vi "resolve control references.vi"(4 "output dictionary":refnum<class "data dictionary.lvclass">, 6 "input dictionary":refnum<class "data dictionary.lvclass">, 8 "error in":errorcluster, 10 "bitfile ref":refnum<k20>, 11 "channels in":refnum<class "TBM channel.lvclass">[](array[class])) -> (0 "error out":errorcluster, 2 "indicators":T1[](array[typedef]), 3 "controls":T1[](array[typedef]))   [LabVIEW 2015, in "io runtime.lvclass"]
uses:
  io runtime.lvclass
  <vilib>/NI/Tag Bus Module Framework/channel/TBM channel.lvclass
  control index set.ctl
  <vilib>/NI/Tag Bus/tag/Data Type.ctl
  configuration/fpga resource supported data types.ctl
  <vilib>/NI/Tag Bus/dictionary/data dictionary.lvclass
  fpga channel/fpga channel.lvclass
  <vilib>/NI/Tag Bus Module Framework/channel/TBM channel.lvclass/TBM channel.ctl
  <vilib>/NI/Tag Bus/tag/tag descriptor.lvclass/tag descriptor.ctl
  <vilib>/NI/Tag Bus Module Framework/channel/Read channel classification.vi
  <vilib>/NI/Tag Bus/tag/read tag name.vi
  <vilib>/NI/Tag Bus/tag/read data type.vi
  <vilib>/NI/Tag Bus/tag/tag descriptor.lvclass
  <vilib>/NI/Configuration Framework/NISE_CEF_TreeControl.lvlib
  configuration/io configuration.lvclass
  <vilib>/NI/LVFPGA Adv Session Resources/LVFPGAAdvSessionResources.lvlib
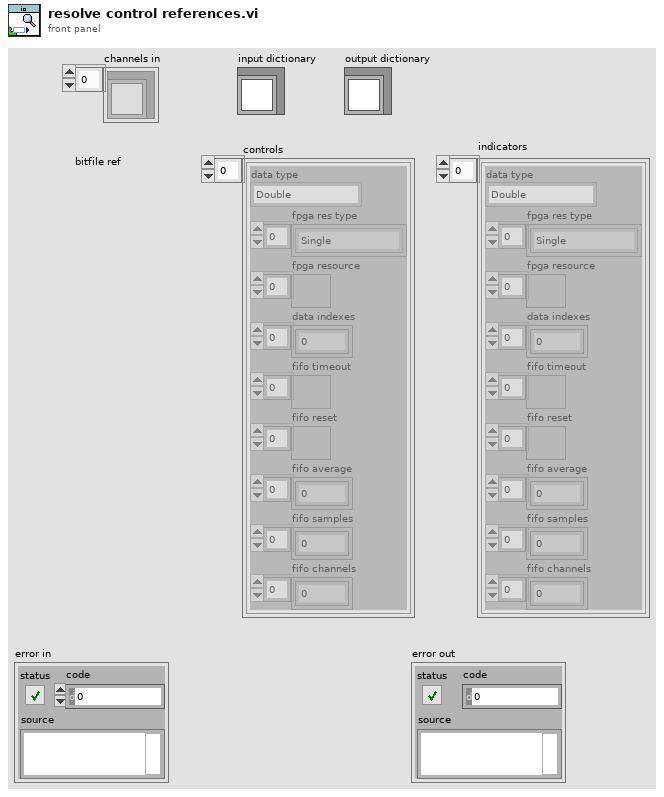
[diagram p1: front panel]
types:
  T1 = typedef "io runtime.lvclass/control index set.ctl" = cluster{"data type":T2, "fpga res type":T3[], "fpga resource":refnum<k20>[], "data indexes":i32[], "fifo timeout":refnum<k20>[], "fifo reset":refnum<k20>[], "fifo average":i32[], "fifo samples":u32[], "fifo channels":u32[]}
  T2 = typedef "tag bus.lvlib/tag descriptor.lvclass/Data Type.ctl" = enum16{"Double", "Single", "I64", "I32", "I16", "I8", "U64", "U32", "U16", "U8", "Boolean", "String", "Array of Double", "Array of Single", "Array of I64", "Array of I32", "Array of I16", "Array of I8", "Array of U64", "Array of U32", "Array of U16", "Array of U8", "Array of Boolean", "Array of String"}
  T3 = typedef "io configuration.lvclass/fpga resource supported data types.ctl" = enum16{"Invalid Type", "Single", "I64", "I32", "I16", "I8", "U64", "U32", "U16", "U8", "Boolean", "FXP I,20,5", "FXP I,24,5", "FXP I,24,10", "Fifo 1023,I16"}
  T4 = typedef "LVFPGAAdvSessionResources.lvlib/ResourceInfo.ctl" = cluster{"Resource name":string, "Data type":variant, "Resource type":enum16{"Register", "Host To Target FIFO", "Target To Host FIFO"}}
  T5 = typedef "TBM channel.lvclass/channel classification.ctl" = enum16{"input data", "output data", "processing parameter", "processing result"}
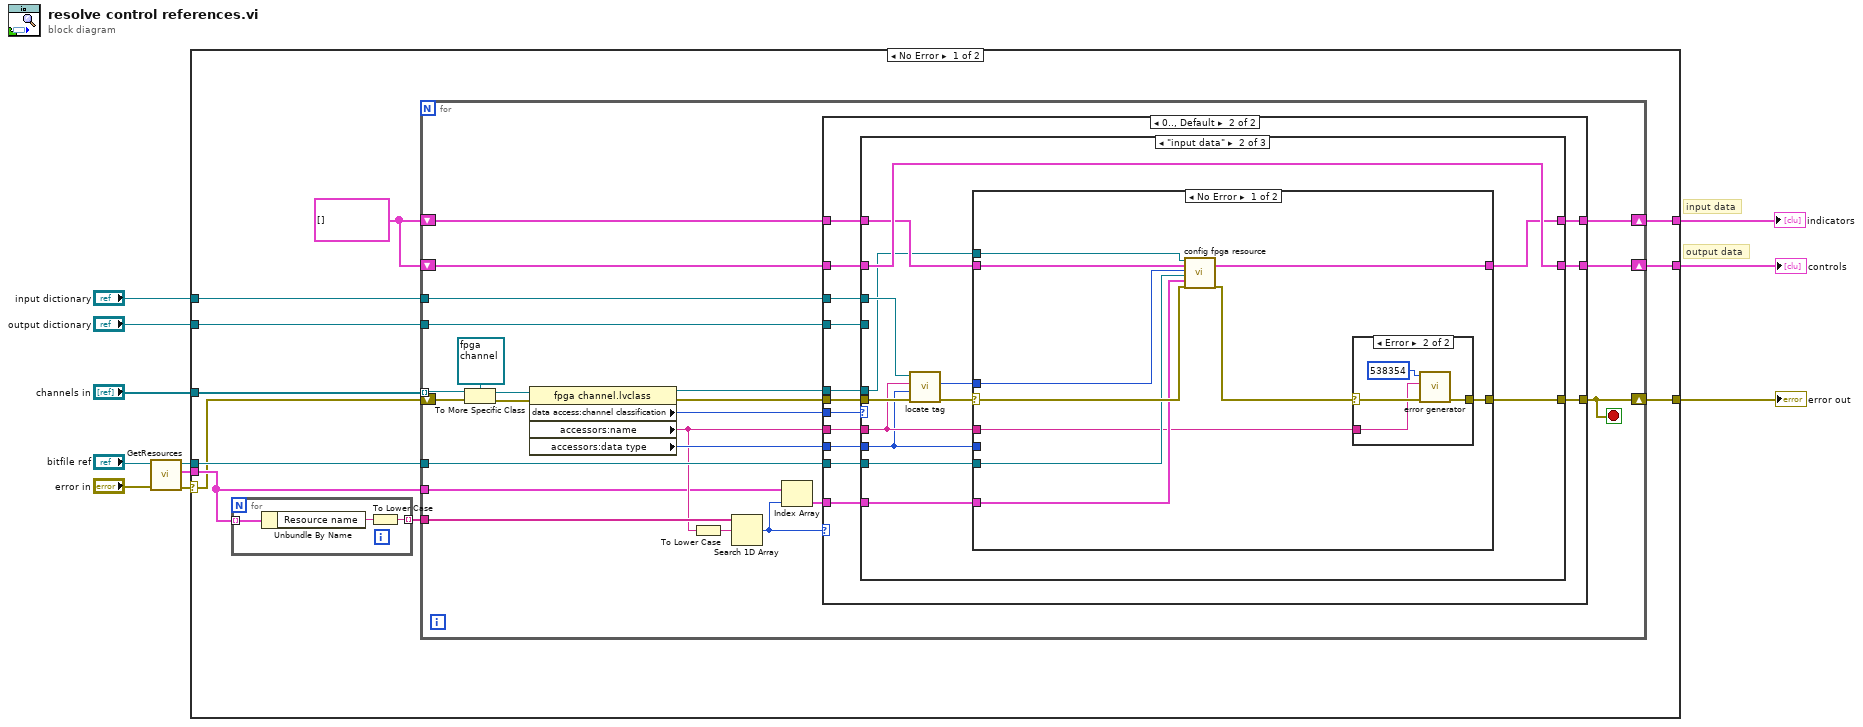
[diagram p0: block diagram]
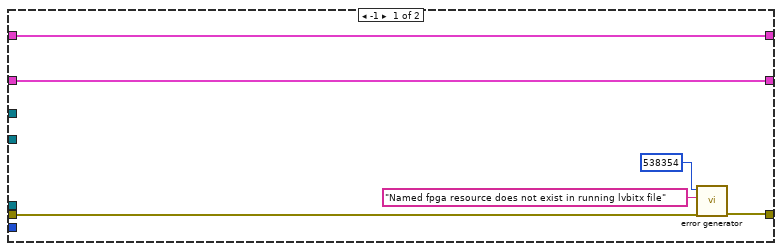
[diagram p2: hidden frame]
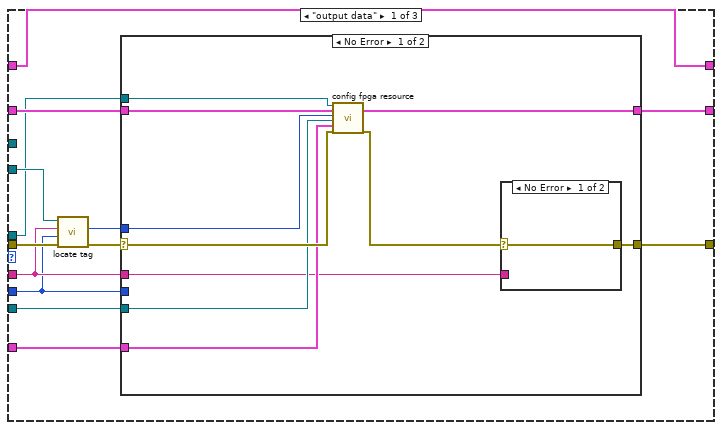
[diagram p3: hidden frame]
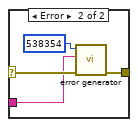
[diagram p4: hidden frame]
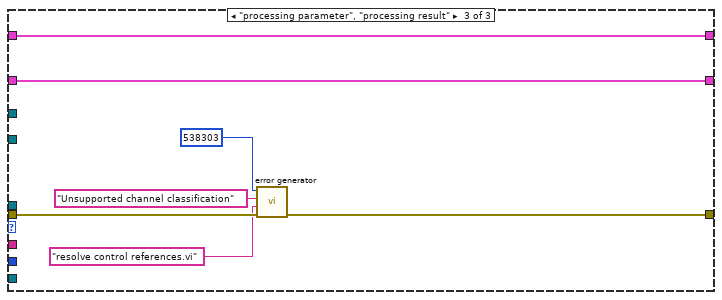
[diagram p8: hidden frame]
diagram:
  # "input data"
  # "output data"
  n1 = call <vilib>:"GetResources.vi"("error in (no error)"="error in", "FPGA VI Reference in"="bitfile ref") -> ("error out"=w1:errorcluster, "Resource info out"=w2:T4[], "FPGA VI Reference out"=w3:refnum<k20>)  [unwired: 7 in]
  n2 = case shown="No Error" w1 {
    selector: w1 -> [w12 w136]
    tunnel: "channels in" -> [w22 _]
    tunnel: [w20 _] -> w6
    tunnel: [w19 _] -> w5
    tunnel: "output dictionary" -> [w18 _]
    tunnel: "input dictionary" -> [w17 _]
    tunnel: [w16 w136] -> w7
    tunnel: w3 -> [w14 _]
    tunnel: w2 -> [w13 _]
    frame No Error {
      w21 = T1[] [] ("indicators")
      n3 = for {
        tunnel: w13 -> [w25] mode=indexing
        tunnel: [w23] -> w15 mode=indexing
        n4 = Unbundle By Name(w25) -> ("Resource name"=w24:string)
        n5 = To Lower Case(string=w24) -> (all lower case string=w23:string)
      }
      n6 = for {
        tunnel: w22 -> [w26] mode=indexing
        shift-right: [w45] -> w20
        shift-left: w21 -> [w44]
        shift-right: [w42] -> w19
        shift-left: w21 -> [w43]
        shift-right: [w46] -> w16
        shift-left: w12 -> [w33]
        tunnel: w18 -> [w40]
        tunnel: w17 -> [w41]
        tunnel: w14 -> [w39]
        tunnel: w15 -> [w36]
        tunnel: w13 -> [w29]
        stop <- w46 stop-if-true
        n7 = To More Specific Class(target class=refnum<class "fpga channel.lvclass"> refnum ("fpga channel.lvclass"), reference=w26, error in=w33) -> (specific class reference=w32:refnum<class "fpga channel.lvclass">, error out=w27:errorcluster)
        n8 = property class="fpga channel.lvclass"(reference=w32, error in=w27) -> (reference out=w37:refnum<class "fpga channel.lvclass">, error out=w47:errorcluster, "data access:channel classification"=w48:T5, "accessors:name"=w35:string, "accessors:data type"=w38:T2)
        n9 = To Lower Case(string=w35) -> (all lower case string=w34:string)
        n10 = Search 1D Array(1D array=w36, element=w34) -> (index of element=w30:i32)  [unwired: 1 in]
        n11 = Index Array(array=w29, index=w30) -> (element=w28:T4)
        n12 = case shown="0.., Default" w30 {
          tunnel: w48 -> [_ w68]
          tunnel: w47 -> [w53 w67]
          tunnel: [w52 w66] -> w46
          tunnel: [w51 w65] -> w45
          tunnel: w44 -> [w51 w64]
          tunnel: w43 -> [w50 w63]
          tunnel: [w50 w62] -> w42
          tunnel: w41 -> [_ w61]
          tunnel: w40 -> [_ w60]
          tunnel: w39 -> [_ w59]
          tunnel: w38 -> [_ w58]
          tunnel: w37 -> [_ w57]
          tunnel: w35 -> [_ w56]
          tunnel: w28 -> [_ w55]
          frame -1 {
            n13 = call <vilib>:"error generator.vi"("error in"=w53, "append error message"="Named fpga resource does not exist in running lvbitx file", "error code (0)"=538354) -> ("error out"=w52:errorcluster)  [unwired: 6 in]
          }
          frame 0.., Default {
            n14 = case shown="\"input data\"" w68 {
              tunnel: w67 -> [w81 w110 w135]
              tunnel: [w77 w106 w133] -> w66
              tunnel: [w71 w100 w130] -> w65
              tunnel: w64 -> [w71 w101 w130]
              tunnel: w63 -> [w73 w111 w129]
              tunnel: [w72 w111 w129] -> w62
              tunnel: w61 -> [_ w102 _]
              tunnel: w56 -> [w79 w108 _]
              tunnel: w58 -> [w78 w107 _]
              tunnel: w60 -> [w74 _ _]
              tunnel: w59 -> [w75 w104 _]
              tunnel: w57 -> [w70 w99 _]
              tunnel: w55 -> [w69 w103 _]
              frame "output data" {
                n15 = call <vilib>:"locate tag.vi"("error in"=w81, "data type"=w78, "name"=w79, "data dictionary in"=w74) -> ("error out"=w80:errorcluster, "index"=w76:i32)  [unwired: 5 in, 1 out]
                n16 = case shown="No Error" w80 {
                  selector: w80 -> [w90 w98]
                  tunnel: w79 -> [w82 _]
                  tunnel: w78 -> [_ _]
                  tunnel: [w91 w98] -> w77
                  tunnel: w73 -> [w87 w97]
                  tunnel: [w86 w97] -> w72
                  tunnel: w76 -> [w85 _]
                  tunnel: w75 -> [w84 _]
                  tunnel: w70 -> [w88 _]
                  tunnel: w69 -> [w83 _]
                  frame No Error {
                    n17 = call-dynamic "config fpga resource.vi"("fpga channel in"=w88, "pairs in"=w87, "tagbus index"=w85, "bitfile ref in"=w84, "hardware resource"=w83, "error in (no error)"=w90) -> ("pairs out"=w86:T1[], "error out"=w89:errorcluster)  [unwired: 11 in, 1 out]
                    n18 = case shown="No Error" w89 {
                      selector: w89 -> [w92 w94]
                      tunnel: [w92 w95] -> w91
                      tunnel: w82 -> [_ w93]
                      frame No Error {
                      }
                      frame Error {
                        n19 = call <vilib>:"error generator.vi"("error in"=w94, "append error message"=w93, "error code (0)"=538354) -> ("error out"=w95:errorcluster)  [unwired: 6 in]
                      }
                    }
                  }
                  frame Error {
                  }
                }
              }
              frame "input data" {
                n20 = call <vilib>:"locate tag.vi"("error in"=w110, "data type"=w107, "name"=w108, "data dictionary in"=w102) -> ("error out"=w109:errorcluster, "index"=w105:i32)  [unwired: 5 in, 1 out]
                n21 = case shown="No Error" w109 {
                  selector: w109 -> [w120 w128]
                  tunnel: w108 -> [w112 _]
                  tunnel: w107 -> [_ _]
                  tunnel: [w121 w128] -> w106
                  tunnel: w101 -> [w117 w127]
                  tunnel: [w116 w127] -> w100
                  tunnel: w105 -> [w115 _]
                  tunnel: w104 -> [w114 _]
                  tunnel: w99 -> [w118 _]
                  tunnel: w103 -> [w113 _]
                  frame No Error {
                    n22 = call-dynamic "config fpga resource.vi"("fpga channel in"=w118, "pairs in"=w117, "tagbus index"=w115, "bitfile ref in"=w114, "hardware resource"=w113, "error in (no error)"=w120) -> ("pairs out"=w116:T1[], "error out"=w119:errorcluster)  [unwired: 11 in, 1 out]
                    n23 = case shown="Error" w119 {
                      selector: w119 -> [w122 w124]
                      tunnel: [w122 w125] -> w121
                      tunnel: w112 -> [_ w123]
                      frame No Error {
                      }
                      frame Error {
                        n24 = call <vilib>:"error generator.vi"("error in"=w124, "append error message"=w123, "error code (0)"=538354) -> ("error out"=w125:errorcluster)  [unwired: 6 in]
                      }
                    }
                  }
                  frame Error {
                  }
                }
              }
              frame "processing parameter", "processing result" {
                n25 = call <vilib>:"error generator.vi"("error in"=w135, "source"="resolve control references.vi", "append error message"="Unsupported channel classification", "error code (0)"=538303) -> ("error out"=w133:errorcluster)  [unwired: 5 in]
              }
            }
          }
        }
      }
    }
    frame Error {
    }
  }
  "controls" <- w5
  "indicators" <- w6
  "error out" <- w7
